vi "CLD 4 Event Structure Time Out Front Panel.vi"() -> ()   [LabVIEW 2017]
doc: "CLD 4 exercise"
panel:
  out "Count":i32
  in  "Decrement":bool
  out "Error Out":errorcluster
  in  "Error In":errorcluster
  out "Time Has Elapsed":bool
  in  "Increment":bool
  in  "Stop VI":bool
  in  "Timeout Target (s)":dbl=2.0
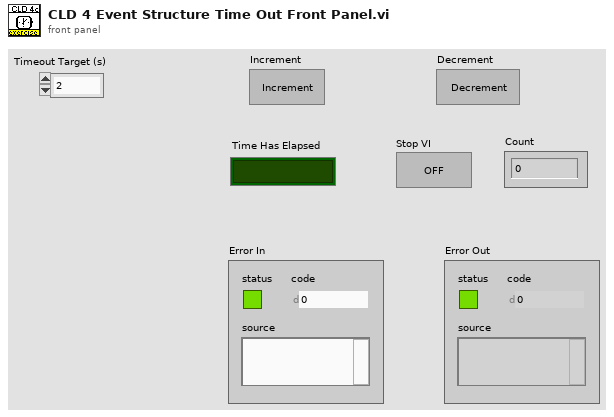
[diagram p1: front panel]
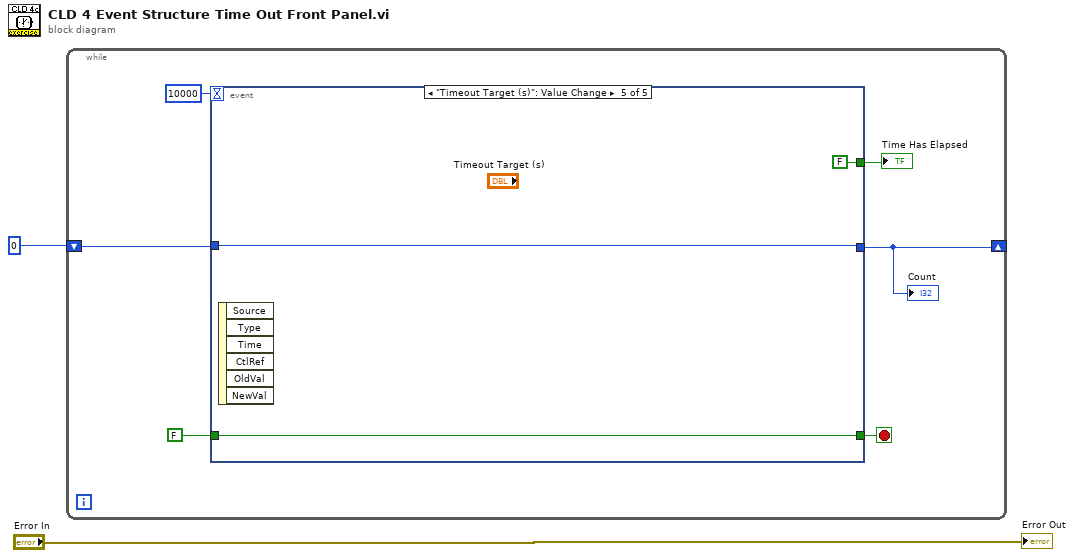
[diagram p0: block diagram]
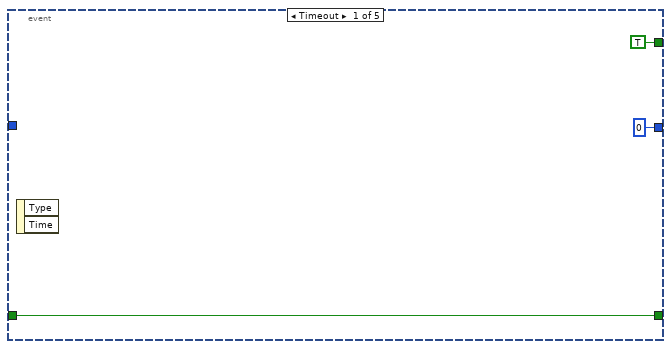
[diagram p2: hidden frame]
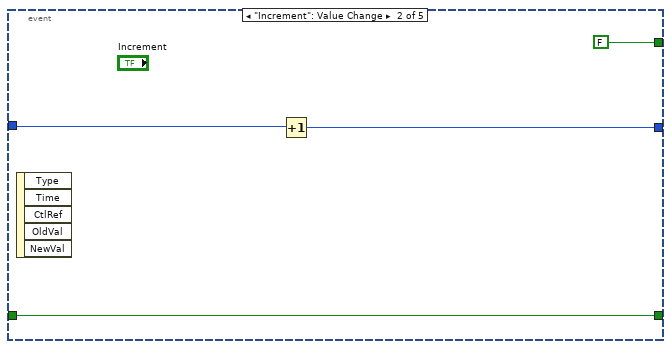
[diagram p3: hidden frame]
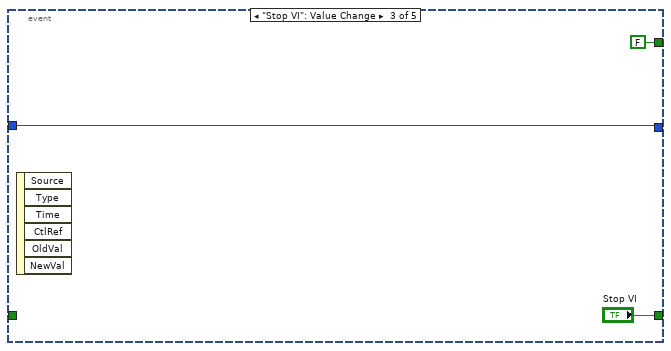
[diagram p4: hidden frame]
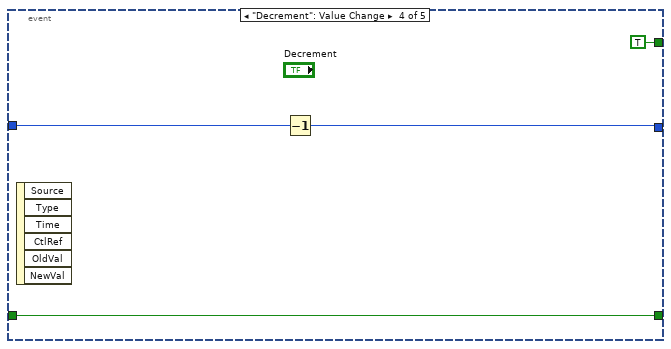
[diagram p5: hidden frame]
diagram:
  n1 = while {
    shift-right: [w6] -> _
    shift-left: 0 -> [w7]
    stop <- w5 stop-if-true
    n2 = event shown="[4] \"Timeout Target (s)\": Value Change" {
      selector: _ -> [_ _ _ _ _]
      dyn-events: _ -> [_ _ _ _ _]
      timeout: 10000 -> [_ _ _ _ _]
      tunnel: [TRUE FALSE FALSE TRUE FALSE] -> w8
      tunnel: w7 -> [_ w14 w16 w20 w24]
      tunnel: [0 w13 w16 w19 w24] -> w6
      tunnel: [w11 w12 "Stop VI" w22 w25] -> w5
      tunnel: FALSE -> [w11 w12 _ w22 w25]
      event Timeout {
        n3 = event-data() -> ()  [unwired: 1 in, 2 out]
      }
      event "Increment": Value Change {
        n4 = event-data() -> ()  [unwired: 1 in, 5 out]
        n5 = Increment(x=w14) -> (x+1=w13:i32)
      }
      event "Stop VI": Value Change {
        n6 = event-data() -> ()  [unwired: 1 in, 6 out]
      }
      event "Decrement": Value Change {
        n7 = event-data() -> ()  [unwired: 1 in, 6 out]
        n8 = Decrement(x=w20) -> (x-1=w19:i32)
      }
      event "Timeout Target (s)": Value Change {
        n9 = event-data() -> ()  [unwired: 1 in, 6 out]
      }
    }
    "Time Has Elapsed" <- w8
    "Count" <- w6
  }
  "Error Out" <- "Error In"
